vi "CMD_MOVESAFE.vi"(6 "Gantry in":refnum<class "Gantry.lvclass">, 8 "error in (no error)":errorcluster, 10 "Arguments":string[](array[string]), 11 "gScript Interpreter in":refnum<class "gScript Interpreter.lvclass">) -> (0 "error out":errorcluster, 3 "gScript Interpreter out":refnum<class "gScript Interpreter.lvclass">, 4 "Gantry out":refnum<class "Gantry.lvclass">)   [LabVIEW 2017, in "gScript Interpreter.lvclass"]
uses:
  gScript Interpreter.lvclass
  Shared Components/Gantry Class/Gantry.lvclass
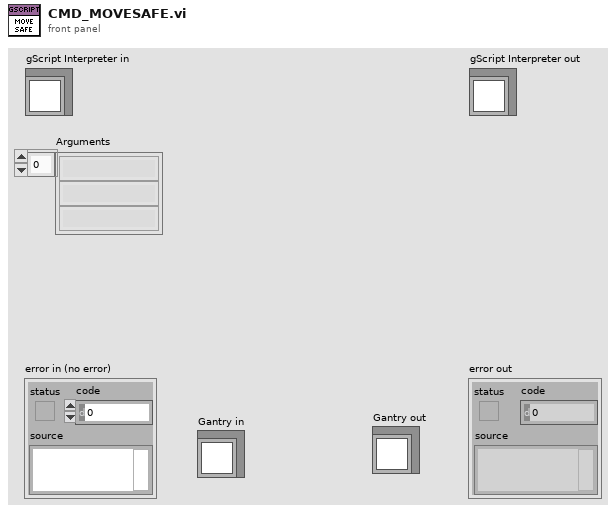
[diagram p1: front panel]
types:
  T1 = enum16{"Vertical First", "Lateral First", "Auto"}
  T2 = typedef "Memory Cell.ctl" = cluster{"type":T3, "x":dbl, "y":dbl, "z":dbl, "w":dbl}
  T3 = typedef "Memory Cell Type Enum.ctl" = enum16{"integer", "float", "vector", "rotation"}
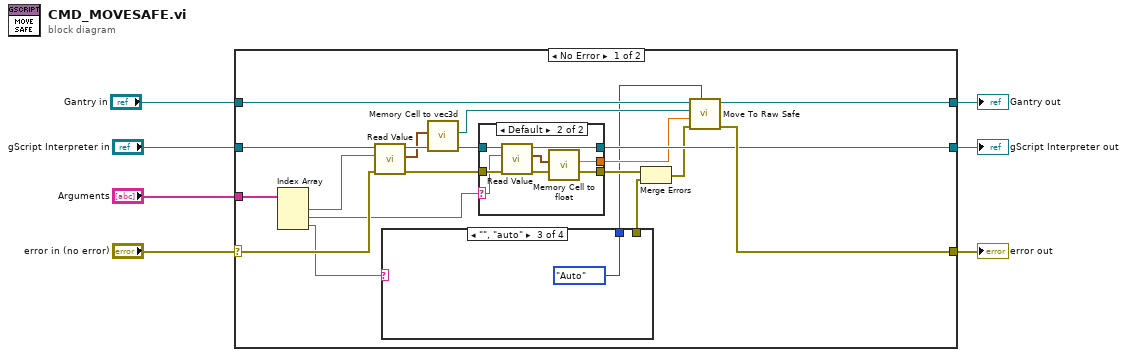
[diagram p0: block diagram]
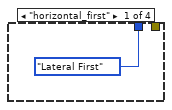
[diagram p2: hidden frame]
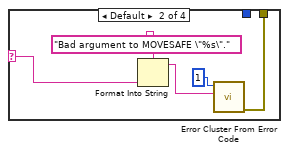
[diagram p3: hidden frame]
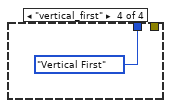
[diagram p4: hidden frame]
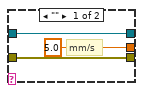
[diagram p5: hidden frame]
diagram:
  n1 = case shown="No Error" "error in (no error)" {
    selector: "error in (no error)" -> [w22 w47]
    tunnel: [w24 w47] -> w6
    tunnel: [w15 w46] -> w4
    tunnel: "gScript Interpreter in" -> [w23 w46]
    tunnel: "Arguments" -> [w21 _]
    tunnel: "Gantry in" -> [w26 w45]
    tunnel: [w25 w45] -> w1
    frame No Error {
      n2 = Index Array(array=w21) -> (element #1=w20:string, element #2=w13:string, element #3=w12:string)  [unwired: 3 in]
      n3 = call-dynamic "Read Value.vi"("error in (no error)"=w22, "String in"=w20, "gScript Interpreter in"=w23) -> ("error out"=w18:errorcluster, "Memory Cell"=w17:T2, "gScript Interpreter out"=w19:refnum<class "gScript Interpreter.lvclass">)  [unwired: 6 in]
      n4 = case shown="\"\", \"auto\"" w12 {
        selector: w12 -> [_ w29 _ _]
        tunnel: [_ w31 _ _] -> w9
        tunnel: [T1."Lateral First" ("Motion Order") _ T1."Auto" ("Motion Order") T1."Vertical First" ("Motion Order")] -> w8
        frame "horizontal_first" {
        }
        frame Default {
          n5 = Format Into String(format string="Bad argument to MOVESAFE \"%s\"." ("error message (\"\")"), w29) -> (resulting string=w28:string)  [unwired: 2 in, 1 out]
          n6 = call <vilib>:"Error Cluster From Error Code.vi"("error message (\"\")"=w28, "error code (0)"=1) -> ("error out"=w31:errorcluster)  [unwired: 7 in]
        }
        frame "", "auto" {
        }
        frame "vertical_first" {
        }
      }
      n7 = call "Memory Cell to vec3d.vi"("Memory Cell"=w17) -> ("Vec3d out"=w16:refnum<class "Vec3d.lvclass">)  [unwired: 10 in]
      n8 = case shown="Default" w13 {
        selector: w13 -> [_ w39]
        tunnel: w19 -> [w37 w44]
        tunnel: w18 -> [w36 w43]
        tunnel: [w37 w42] -> w15
        tunnel: [5.0 ("float out") w40] -> w14
        tunnel: [w36 w38] -> w11
        frame "" {
          # "mm/s"
        }
        frame Default {
          n9 = call-dynamic "Read Value.vi"("error in (no error)"=w43, "String in"=w39, "gScript Interpreter in"=w44) -> ("error out"=w38:errorcluster, "Memory Cell"=w41:T2, "gScript Interpreter out"=w42:refnum<class "gScript Interpreter.lvclass">)  [unwired: 6 in]
          n10 = call "Memory Cell to float.vi"("Memory Cell"=w41) -> ("float out"=w40:dbl)  [unwired: 10 in]
        }
      }
      n11 = Merge Errors(w11, w9) -> (w10:errorcluster)
      n12 = call-dynamic "Move To Raw Safe.vi"("Motion Order"=w8, "error in"=w10, "Speed(mm/s)"=w14, "Destination"=w16, "Gantry in"=w26) -> ("error out"=w24:errorcluster, "Gantry out"=w25:refnum<class "Gantry.lvclass">)  [unwired: 5 in]
    }
    frame Error {
    }
  }
  "error out" <- w6
  "gScript Interpreter out" <- w4
  "Gantry out" <- w1
